vi "CCC.vi"(0 "comm interface in":refnum<class "Pixy Com.lvclass">, 5 "signature map":u8=255 format="%.0b", 7 "max blocks":u8=255, 11 "error in":errorcluster) -> (4 "comm interface out":refnum<class "Pixy Com.lvclass">, 6 "blocks":T1[](array[typedef]), 15 "error out":errorcluster)   [LabVIEW 2018, in "Pixy2.lvlib"]
uses:
  Pixy2.lvlib
  Interface/Pixy Com.lvclass
  Types/Block.ctl
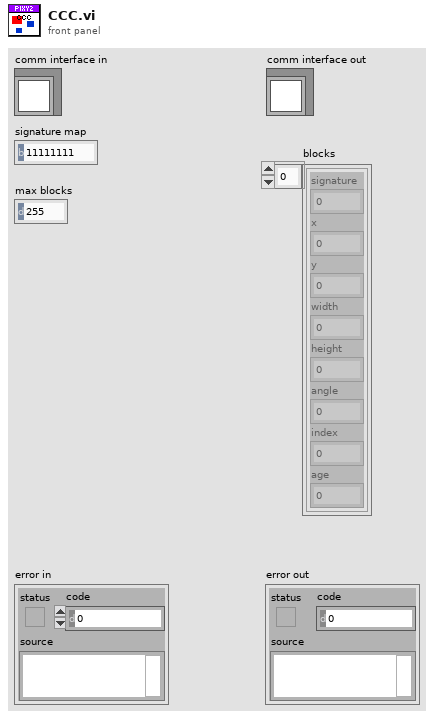
[diagram p1: front panel]
types:
  T1 = typedef "Pixy2.lvlib/Block.ctl" = cluster{"signature":u16, "x":u16, "y":u16, "width":u16, "height":u16, "angle":i16, "index":u8, "age":u8}
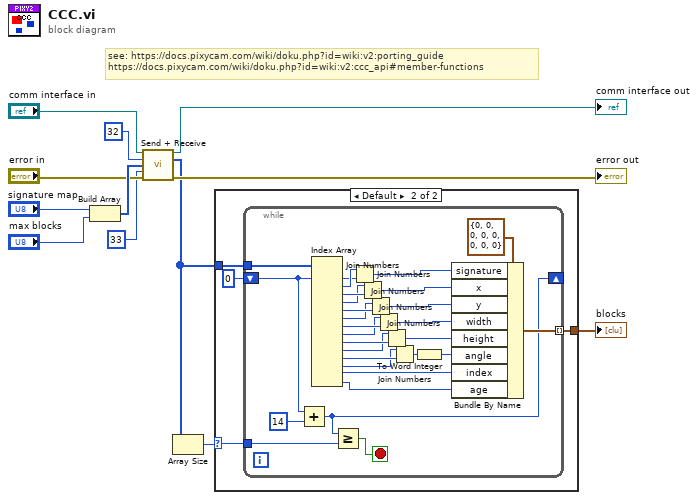
[diagram p0: block diagram]
diagram:
  # "see: https://docs.pixycam.com/wiki/doku.php?id=wiki:v2:porting_guide\nhttps://docs.pixycam.com/wiki/doku.php?id=wiki:v2:ccc_api#member-functions"
  n1 = Build Array("signature map", "max blocks") -> (w4:u8[])
  n2 = call "Send + Receive.vi"("comm interface in"="comm interface in", "type"=u8 32, "payload"=w4, "expected response"=u8 33 ("type"), "error in"="error in") -> ("comm interface out"=→"comm interface out":refnum<class "Pixy Com.lvclass">, "received"=w7:u8[], "error out"=→"error out":errorcluster)  [unwired: 8 in]
  n3 = Array Size(array=w7) -> (size(s)=w6:i32)
  n4 = case shown="Default" w6 {
    selector: w6 -> [_ w13]
    tunnel: [_ w16] -> w8
    tunnel: w7 -> [_ w14]
    frame 0 {
    }
    frame Default {
      n5 = while {
        tunnel: [w22] -> w16 mode=indexing
        shift-right: [w18] -> _
        shift-left: 0 -> [w21]
        tunnel: w14 -> [w45]
        tunnel: w13 -> [w19]
        stop <- w17 stop-if-true
        n6 = Add(x=w21, y=14) -> (x+y=w18:i32)
        n7 = Index Array(array=w45, index #1=w21) -> (element #1=w42:u8, element #2=w43:u8, element #3=w41:u8, element #4=w40:u8, element #5=w37:u8, element #6=w36:u8, element #7=w35:u8, element #8=w34:u8, element #9=w33:u8, element #10=w32:u8, element #11=w28:u8, element #12=w27:u8, element #13=w24:u8, element #14=w23:u8)  [unwired: 13 in]
        n8 = Greater Or Equal?(x=w18, y=w19) -> (x >= y?=w17:bool)
        n9 = Join Numbers(hi=w43, lo=w42) -> ((hi.lo)=w39:u16)
        n10 = Join Numbers(hi=w40, lo=w41) -> ((hi.lo)=w38:u16)
        n11 = Join Numbers(hi=w36, lo=w37) -> ((hi.lo)=w31:u16)
        n12 = Join Numbers(hi=w34, lo=w35) -> ((hi.lo)=w30:u16)
        n13 = Join Numbers(hi=w32, lo=w33) -> ((hi.lo)=w29:u16)
        n14 = Join Numbers(hi=w27, lo=w28) -> ((hi.lo)=w26:u16)
        n15 = To Word Integer(number=w26) -> (16bit integer=w25:i16)
        n16 = Bundle By Name(cluster=T1 {"signature"=0, "x"=0, "y"=0, "width"=0, "height"=0, "angle"=0, "index"=0, "age"=0} ("block"), "signature"=w39, "x"=w38, "y"=w31, "width"=w30, "height"=w29, "angle"=w25, "index"=w24, "age"=w23) -> (w22:T1)
      }
    }
  }
  "blocks" <- w8
